vi "laser power voltage value tester.vi"() -> ()   [LabVIEW 2020]
uses:
  Typedefs/Functional global standard states.ctl
panel:
  out "Back-aperture power (mW)":dbl format="%#_gmW"
  out "Power after the objective (mW)":dbl
  out "Pockels Volts":dbl format="%#_6fV"
  out "Pockels calibration data (Single wavelength)":dbl[][](array[numeric])
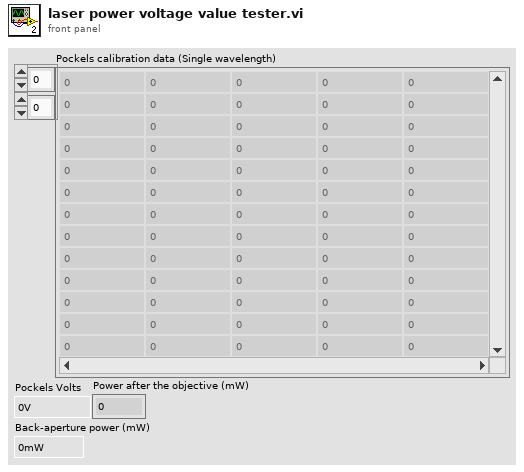
[diagram p1: front panel]
types:
  T1 = typedef "Functional global standard states.ctl" = enum16{"Initialise", "Read", "Write", "Load", "Save", "Clear"}
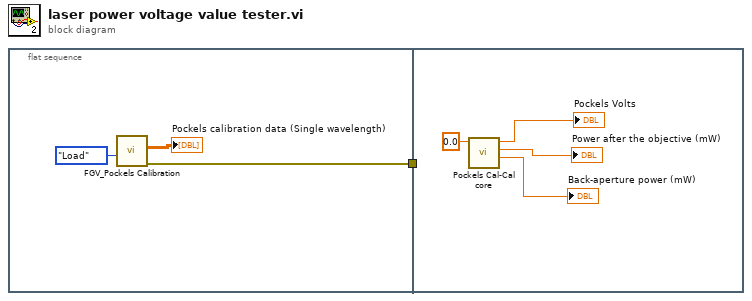
[diagram p0: block diagram]
diagram:
  n1 = flat-sequence {
    tunnel: [w3] -> w1
    tunnel: w1 -> [_]
    frame #0 {
      n2 = call "FGV_Pockels Calibration.vi"("Function"=Functional_global_standard_states."Load") -> ("error out"=w3:errorcluster, "Pockels calibration data (Single wavelength)"=→"Pockels calibration data (Single wavelength)":dbl[][])  [unwired: 4 in, 5 out]
    }
    frame #1 {
      n3 = call "Pockels Cal-Cal core.vi"("Pockels power (%)"=0.0) -> ("Back-aperture power (mW)"=→"Back-aperture power (mW)":dbl, "Power after the objective (mW)"=→"Power after the objective (mW)":dbl, "Pockels Volts"=→"Pockels Volts":dbl)  [unwired: 8 in]
    }
  }
